vi "scope_interface.vi"() -> ()   [LabVIEW 2011]
panel:
  out "error out 2":errorcluster
  in  "error in (no error) 2":errorcluster
  out "error out":errorcluster {"code" format="%.0x"}
  in  "error in (no error)":errorcluster {"code" format="%.0x"}
  out "Scope Data":string
  in  "VISA Scope":refnum<visa-resource-name>
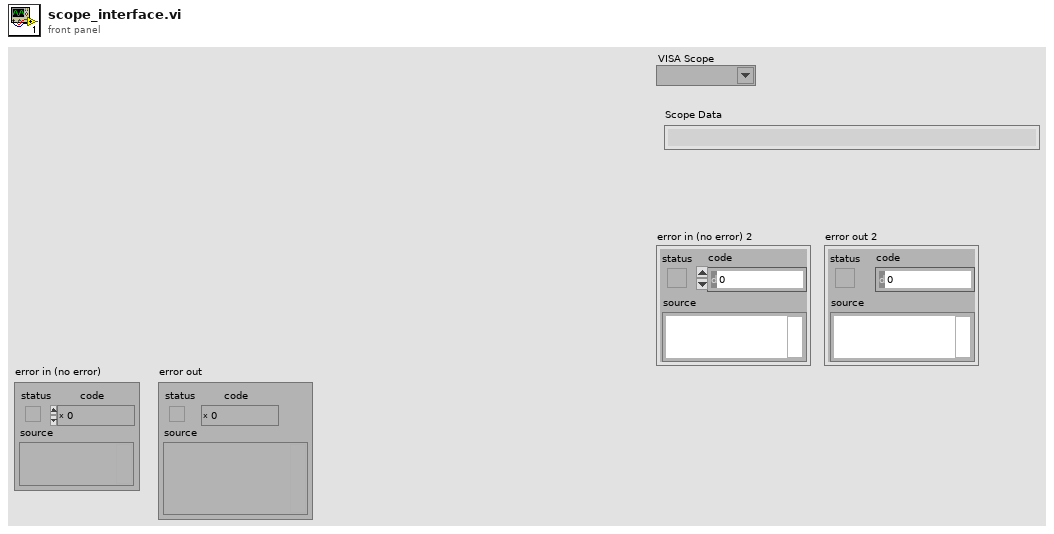
[diagram p1: front panel]
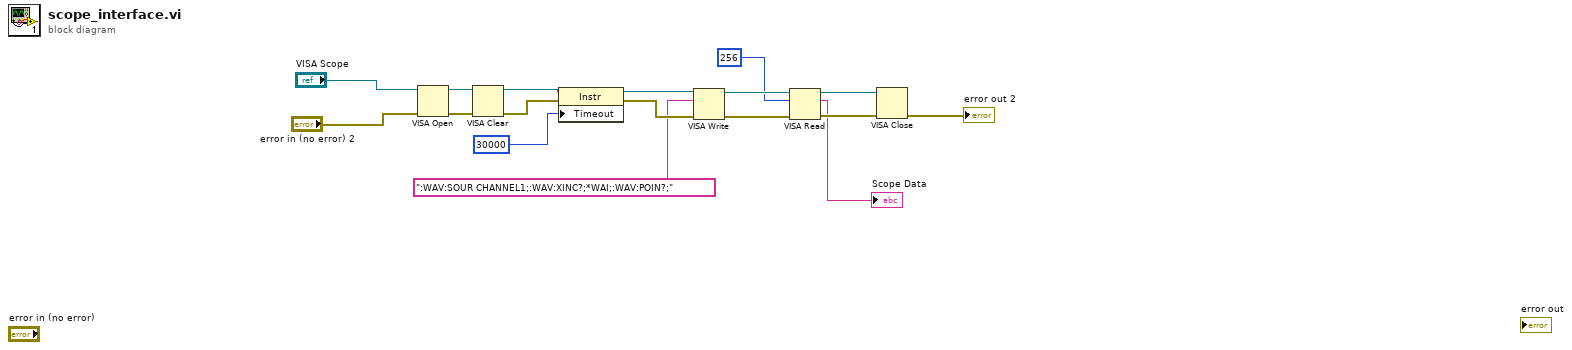
[diagram p0: block diagram]
diagram:
  n1 = VISA Open(error in (no error)="error in (no error) 2", VISA resource name="VISA Scope") -> (VISA resource name=w14:refnum<visa-resource-name>, error out=w15:errorcluster)  [unwired: 3 in]
  n2 = VISA Clear(VISA resource name=w14, error in (no error)=w15) -> (VISA resource name out=w13:refnum<visa-resource-name>, error out=w12:errorcluster)
  n3 = property class="Instr"(reference=w13, error in=w12, "Timeout"=u32 30000 ("General Settings:Timeout Value")) -> (reference out=w10:refnum<visa-resource-name>, error out=w9:errorcluster)
  n4 = VISA Write(VISA resource name=w10, write buffer=":WAV:SOUR CHANNEL1;:WAV:XINC?;*WAI;:WAV:POIN?;", error in (no error)=w9) -> (VISA resource name out=w7:refnum<visa-resource-name>, error out=w6:errorcluster)  [unwired: 1 out]
  n5 = VISA Read(VISA resource name=w7, byte count=u32 256, error in (no error)=w6) -> (VISA resource name out=w3:refnum<visa-resource-name>, read buffer=→"Scope Data":string, error out=w4:errorcluster)  [unwired: 1 out]
  n6 = VISA Close(VISA resource name=w3, error in (no error)=w4) -> (error out=→"error out 2":errorcluster)
